vi "SetupTimedLoop.vi"(8 "error in (no error)":errorcluster, 11 "DaqMx_Single in":refnum<class "DaqMx_Single.lvclass">) -> (0 "error out":errorcluster, 2 "timing source out":string, 3 "DaqMx_Single out":refnum<class "DaqMx_Single.lvclass">)   [LabVIEW 2014, in "FgenPlugins.lvlib" / "DaqMx_Single.lvclass"]
uses:
  DaqMx_Single.lvclass
  NiPxi6733Class/NiPxi6733.lvclass/NiPxi6733.ctl
  DaqMx_Single.lvclass/DaqMx_Single.ctl
  NiPxi6733Class/Accessors/Read Timebase.vi
  NiPxi6733Class/Accessors/Read SampleRate.vi
  Accessors/Write AiSampleClkTask.vi
  <vilib>/DAQmx/create/timing.llb/DAQmx Create Timing Source (Control Loop From Task).vi
  <resource>/objmgr/daqmx.rc
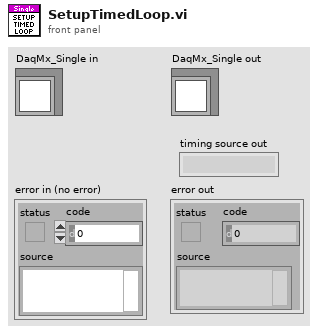
[diagram p1: front panel]
types:
  T1 = typedef "FgenPlugins.lvlib/NiPxi6733.lvclass/Timebase.ctl" = cluster{"source":string, "rate":dbl}
  T2 = typedef "FgenPlugins.lvlib/Channel.ctl" = cluster{"Name":string, "Enabled":bool, "Operation":enum16{"Continuous", "Burst"}, "Impedance (50)":dbl, "Handle":string, "Connected":bool, "Mode (Function)":enum16{"Function", "Arbitrary", "Sequence"}}
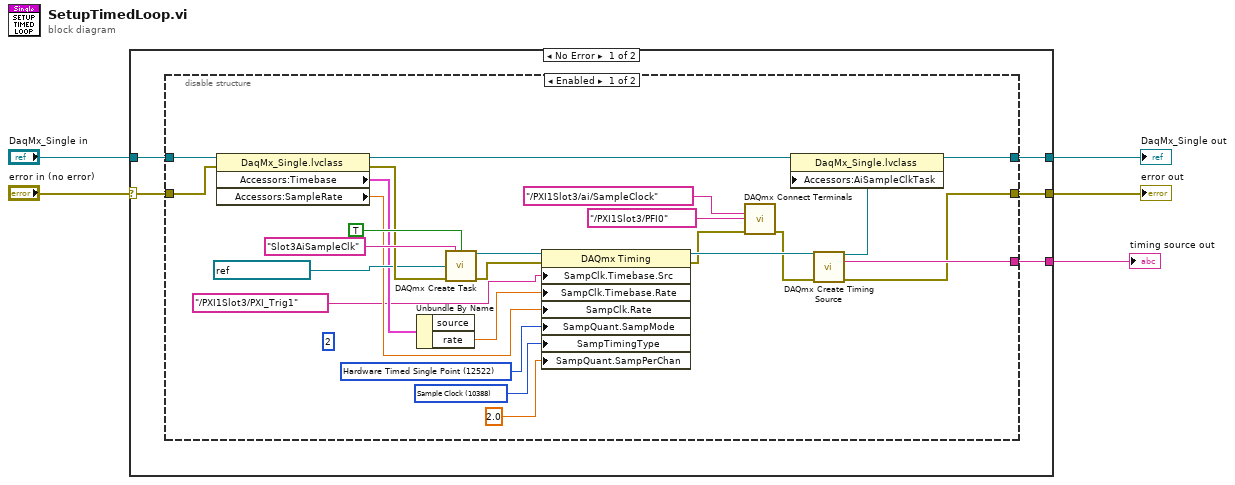
[diagram p0: block diagram]
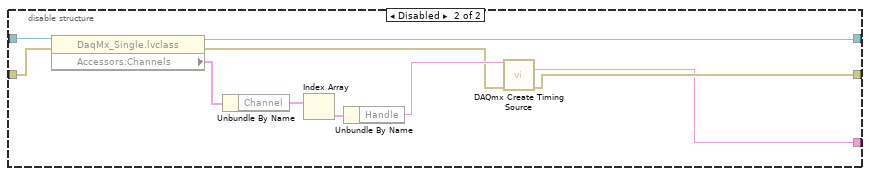
[diagram p2: hidden frame]
diagram:
  n1 = case shown="No Error" "error in (no error)" {
    selector: "error in (no error)" -> [w9 w47]
    tunnel: [w7 w47] -> w4
    tunnel: [w6 w46] -> w2
    tunnel: "DaqMx_Single in" -> [w10 w46]
    tunnel: [w8 _] -> w1
    frame No Error {
      n2 = disable-structure shown="Enabled" {
        disable-tunnel: w10 -> [w35 w45]
        disable-tunnel: w9 -> [w33 w44]
        disable-tunnel: [w32 w36] -> w8
        disable-tunnel: [w31 w38] -> w7
        disable-tunnel: [w27 w37] -> w6
        frame Enabled {
          w19 = 10388 items=["Sample Clock"=10388, "Burst Handshake"=12548, "Handshake"=10389, "Implicit"=10451, "On Demand"=10390, "Change Detection"=12504, "Pipelined Sample Clock"=14668] ("SampTimingType")
          (unwired) 2 ("samples per channel")
          w20 = 12522 items=["Finite Samples"=10178, "Continuous Samples"=10123, "Hardware Timed Single Point"=12522] ("sample mode")
          n3 = property class="DaqMx_Single.lvclass"(reference=w35, error in=w33) -> (reference out=w34:refnum<class "DaqMx_Single.lvclass">, error out=w28:errorcluster, "Accessors:Timebase"=w22:T1, "Accessors:SampleRate"=w21:dbl)
          n4 = Unbundle By Name(w22) -> ("rate"=w12:dbl)  [unwired: 1 out]
          n5 = call <vilib>:"DAQmx Create Task.vi"("new task name"="Slot3AiSampleClk", "auto cleanup"=TRUE, "global virtual channels"=refnum<k21> "PXI1Slot3_ai7", "error in"=w28) -> ("task out"=w24:refnum<k21>, "error out"=w23:errorcluster)  [unwired: 10 in]
          n6 = property class="DAQmx Timing"(reference=w24, error in=w23, "SampClk.Timebase.Src"=tag "/PXI1Slot3/PXI_Trig1" ("source"), "SampClk.Timebase.Rate"=w12, "SampClk.Rate"=w21, "SampQuant.SampMode"=w20, "SampTimingType"=w19, "SampQuant.SampPerChan"=2.0) -> (reference out=w17:refnum<k21>, error out=w16:errorcluster)
          n7 = call <vilib>:"DAQmx Connect Terminals.vi"("source terminal"=tag "/PXI1Slot3/ai/SampleClock", "destination terminal"=tag "/PXI1Slot3/PFI0", "error in"=w16) -> ("error out"=w15:errorcluster)  [unwired: 12 in]
          n8 = call-poly <vilib>:"DAQmx Create Timing Source.vi"("task/channels in"=w17, "error in"=w15) -> ("task out"=w26:refnum<k21>, "timing source out"=w32:string, "error out"=w31:errorcluster)  [unwired: 11 in]
          n9 = property class="DaqMx_Single.lvclass"(reference=w34, "Accessors:AiSampleClkTask"=w26) -> (reference out=w27:refnum<class "DaqMx_Single.lvclass">)  [unwired: 1 in, 1 out]
        }
        frame Disabled {
          n10 = property class="DaqMx_Single.lvclass"(reference=w45, error in=w44) -> (reference out=w37:refnum<class "DaqMx_Single.lvclass">, error out=w39:errorcluster, "Accessors:Channels"=w43:cluster{"Count":u16, "Channel":T2[]})
          n11 = Unbundle By Name(w43) -> ("Channel"=w42:T2[])
          n12 = Index Array(array=w42) -> (element=w41:T2)  [unwired: 1 in]
          n13 = Unbundle By Name(w41) -> ("Handle"=w40:string)
          n14 = call-poly <vilib>:"DAQmx Create Timing Source.vi"("task/channels in"=w40, "error in"=w39) -> ("timing source out"=w36:string, "error out"=w38:errorcluster)  [unwired: 11 in, 1 out]
        }
      }
    }
    frame Error {
    }
  }
  "error out" <- w4
  "DaqMx_Single out" <- w2
  "timing source out" <- w1
